vi "MyInterfaceMethod2.vi"(0 "reference in":refnum<class "IMyInterface2.lvclass">, 5 "error in (no error)":errorcluster) -> (14 "reference out":refnum<class "IMyInterface2.lvclass">, 19 "error out":errorcluster)   [LabVIEW 2020, in "IMyInterface2.lvclass"]
uses:
  IMyInterface2.lvclass
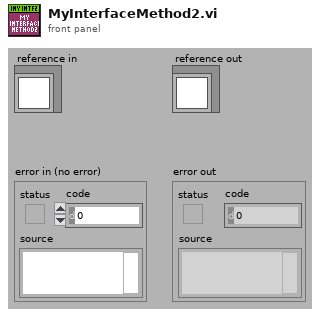
[diagram p1: front panel]
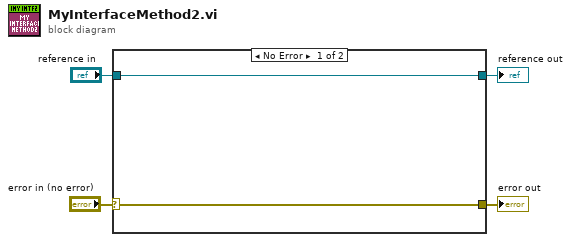
[diagram p0: block diagram]
diagram:
  n1 = case shown="No Error" "error in (no error)" {
    selector: "error in (no error)" -> [w5 w8]
    tunnel: [w5 w8] -> w3
    tunnel: [w6 w7] -> w1
    tunnel: "reference in" -> [w6 w7]
    frame No Error {
    }
    frame Error {
    }
  }
  "error out" <- w3
  "reference out" <- w1
